vi "Update Data Core.vi"(8 "error in":errorcluster, 11 "BNT_DAQmx-MCSV in":refnum<class "BNT_DAQmx-MCSV.lvclass">) -> (0 "error out":errorcluster, 2 "CSPP_DataCollection":refnum<class "CSPP_DataCollection.lvclass">, 3 "BNT_DAQmx-MCSV out":refnum<class "BNT_DAQmx-MCSV.lvclass">)   [LabVIEW 2021, in "BNT_DAQmx.lvlib" / "BNT_DAQmx-MCSV.lvclass"]
doc: "Read data and send to caller actor."
uses:
  BNT_DAQmx-MCSV.lvclass
  CSPP_Core/Classes/CSPP_BaseClasses/DataCollection/CSPP_DataCollection.lvclass
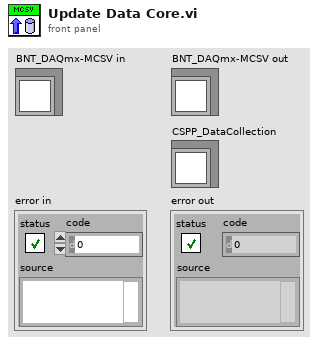
[diagram p1: front panel]
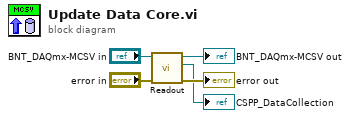
[diagram p0: block diagram]
diagram:
  n1 = call "Readout.vi"("Error In"="error in", "BNT_DAQmx-MCSV in"="BNT_DAQmx-MCSV in") -> ("Error Out"=→"error out":errorcluster, "CSPP_DataCollection out"=→"CSPP_DataCollection":refnum<class "CSPP_DataCollection.lvclass">, "BNT_DAQmx-MCSV out"=→"BNT_DAQmx-MCSV out":refnum<class "BNT_DAQmx-MCSV.lvclass">)  [unwired: 7 in]
